vi "Write EvtConfig.vi"(8 "error in (no error)":errorcluster, 10 "clEvtConfig":T1, 11 "EventPluginBaseClass in":refnum<class "EventPluginBaseClass.lvclass">) -> (0 "error out":errorcluster, 3 "EventPluginBaseClass out":refnum<class "EventPluginBaseClass.lvclass">)   [LabVIEW 2014, in "EventPlugins.lvlib" / "EventPluginBaseClass.lvclass"]
uses:
  EventPluginBaseClass.lvclass
  TypeDefs/clEvtConfig.ctl
  EventPluginBaseClass.lvclass/EventPluginBaseClass.ctl
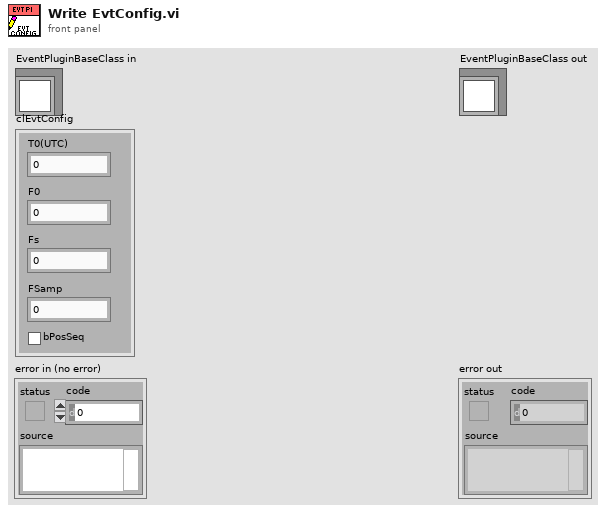
[diagram p1: front panel]
types:
  T1 = typedef "EventPlugins.lvlib/EventPluginBaseClass.lvclass/clEvtConfig.ctl" = cluster{"T0(UTC)":dbl, "F0":dbl, "Fs":i32, "FSamp":u32, "bPosSeq":bool}
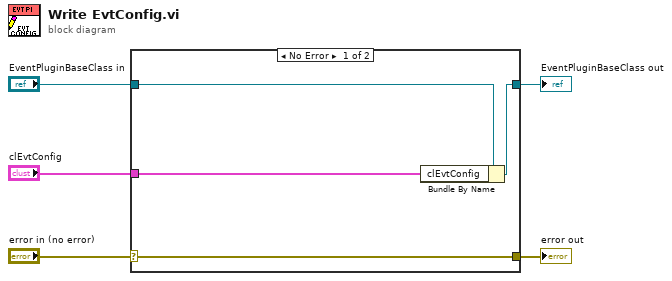
[diagram p0: block diagram]
diagram:
  n1 = case shown="No Error" "error in (no error)" {
    selector: "error in (no error)" -> [w9 w10]
    tunnel: [w9 w10] -> w4
    tunnel: [w7 w11] -> w2
    tunnel: "EventPluginBaseClass in" -> [w8 w11]
    tunnel: "clEvtConfig" -> [w6 _]
    frame No Error {
      n2 = Bundle By Name(cluster=w8, "clEvtConfig"=w6) -> (w7:refnum<class "EventPluginBaseClass.lvclass">)
    }
    frame Error {
    }
  }
  "error out" <- w4
  "EventPluginBaseClass out" <- w2
